vi "Block Name.vi"(8 "error in (no error)":errorcluster, 11 "WaveSourceBlock in":refnum<class "WaveSourceBlock.lvclass">) -> (0 "error out":errorcluster, 2 "Name":string, 3 "WaveSourceBlock out":refnum<class "WaveSourceBlock.lvclass">)   [LabVIEW 2020, in "WaveSourceBlock.lvclass"]
uses:
  WaveSourceBlock.lvclass
  WaveSourceBlock.lvclass/WaveSourceBlock.ctl
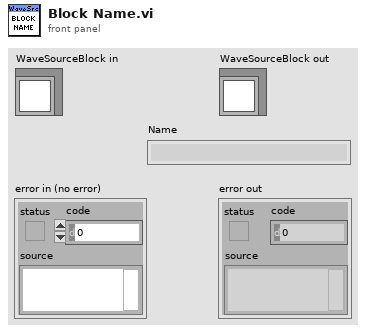
[diagram p1: front panel]
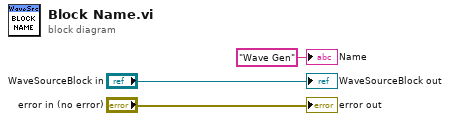
[diagram p0: block diagram]
diagram:
  "error out" <- "error in (no error)"
  "WaveSourceBlock out" <- "WaveSourceBlock in"
  "Name" <- "Wave Gen" ("Name")
